vi "例4.2.vi"() -> ()   [LabVIEW 2018]
panel:
  out "时间":u32
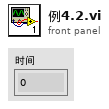
[diagram p1: front panel]
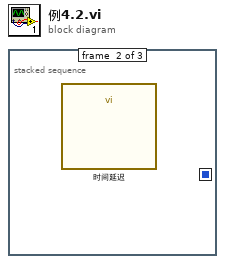
[diagram p0: block diagram]
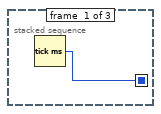
[diagram p2: hidden frame]
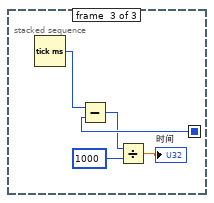
[diagram p3: hidden frame]
diagram:
  n1 = stacked-sequence {
    seq-local: [w1 _ _] -> [_ w2 _]
    seq-local: [_ w2 _] -> [_ _ w6]
    frame #0 {
      n2 = Tick Count (ms)() -> (millisecond timer value=w1:u32)
    }
    frame #1 {
      n3 = call "时间延迟"() -> ()  [unwired: 11 in, 1 out]
    }
    frame #2 {
      n4 = Tick Count (ms)() -> (millisecond timer value=w7:u32)
      n5 = Subtract(x=w7, y=w6) -> (x-y=w5:u32)
      n6 = Divide(x=w5, y=u32 1000) -> (x/y=→"时间":dbl)
    }
  }
